vi "SV UFF58 Format ASCII Function.vi"   [LabVIEW 2017, in "SoundVib_UFF58.lvlib"]
doc: "Formats data to the UFF58 (universal file format) ASCII format. This VI also writes the fields in records 1, 2, and 3, <B>ID lines (1-3)</B> as well as all the records and fields associated with the specified instance and the attributes of input data. You can write a single time domain waveform, a single real frequency spectrum, or a complex frequency spectrum to a UFF58 formatted string. If a frequency spectrum is in decibels, this VI converts the spectrum to linear before writing the data to the formatted string. The default instance, SV UFF58 Format ASCII Function (Time Waveform), writes a single time domain waveform to the file specified by the <B>waveform</B> input. Wire data to the <B>waveform</B> input to determine the polymorphic instance to use or manually select the instance."
uses:
  <vilib>/addons/Sound and Vibration/svt_UFF58/SoundVib_UFF58.lvlib
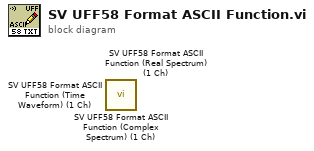
[diagram p0: block diagram]
diagram:
  n1 = call <vilib>:"SV UFF58 Format ASCII Function (Complex Spectrum) (1 Ch).vi"() -> ()  [unwired: 14 in, 2 out]
  n2 = call <vilib>:"SV UFF58 Format ASCII Function (Real Spectrum) (1 Ch).vi"() -> ()  [unwired: 14 in, 2 out]
  n3 = call <vilib>:"SV UFF58 Format ASCII Function (Time Waveform) (1 Ch).vi"() -> ()  [unwired: 14 in, 2 out]
